vi "Get Instrument Path.vi"(8 "error in (no error)":errorcluster, 11 "instrument_type_id":string) -> (0 "error out":errorcluster, 3 "InstrumentClassPath":path)   [LabVIEW 2020, in "Abstract_Instrument.lvlib" / "Abstract_Instrument.lvclass"]
uses:
  Abstract_Instrument.lvclass
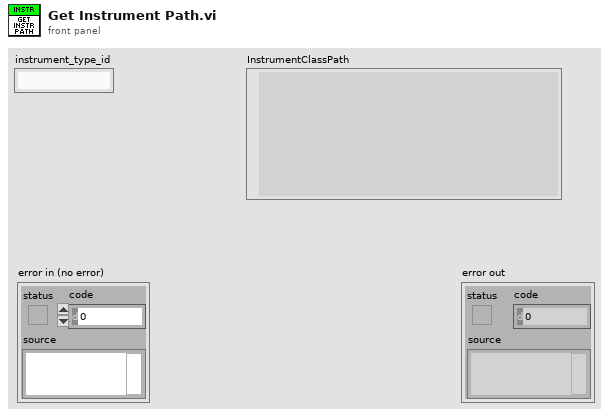
[diagram p1: front panel]
types:
  T1 = typedef "Abstract_Instrument.lvlib/Abstract_Instrument.lvclass/Paths.ctl" = cluster{"InstrumentsClassPath":path}
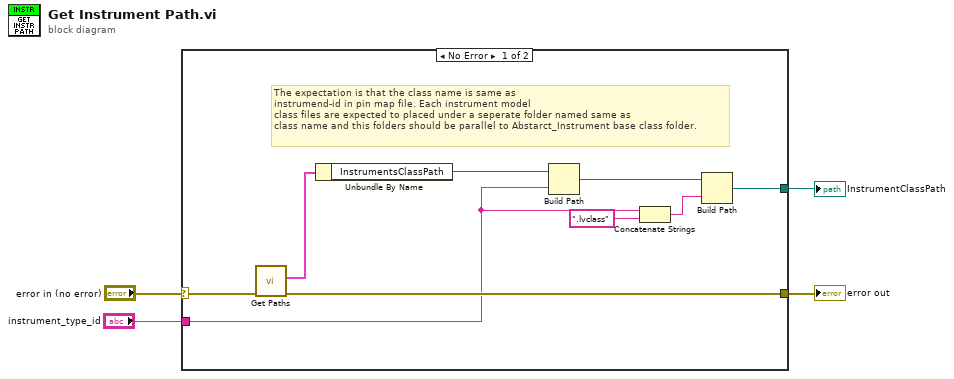
[diagram p0: block diagram]
diagram:
  n1 = case shown="No Error" "error in (no error)" {
    selector: "error in (no error)" -> [w13 w14]
    tunnel: [w12 w14] -> w3
    tunnel: "instrument_type_id" -> [w8 _]
    tunnel: [w5 _] -> w1
    frame No Error {
      # "The expectation is that the class name is same as\ninstrumend-id in pin map file. Each instrument model\nclass files are expected to placed under a seperate folder named same as\nclass name and this folders should be parallel to Abstarct_Instrument base class folder."
      n2 = call "Get Paths.vi"("error in (no error)"=w13) -> ("error out"=w12:errorcluster, "Factory_Paths"=w7:T1)  [unwired: 9 in]
      n3 = Unbundle By Name(w7) -> ("InstrumentsClassPath"=w6:path)
      n4 = Build Path(base path=w6, name or relative path=w8) -> (appended path=w9:path)
      n5 = Concatenate Strings(w8, ".lvclass" ("string")) -> (w10:string)
      n6 = Build Path(base path=w9, name or relative path=w10) -> (appended path=w5:path)
    }
    frame Error {
    }
  }
  "error out" <- w3
  "InstrumentClassPath" <- w1
